vi "Unpack Control Mouse Enter.vi"(11 "ControlMouseEnterMsg":refnum<class "ControlMouseEnterMsg.lvclass">) -> (2 "Time":u32, 3 "Control Label":string, 5 "Ctl Refnum":refnum<vi>)   [LabVIEW 2015, in "ActorEvents.lvlib" / "ControlMouseEnterMsg.lvclass"]
doc: "<License>\nCopyright © 2017 Composed Systems, LLC | All rights reserved\nwww.composed.io\n\nAuthor: Ethan Stern <ethan.stern@composed.io>\n\nThis software is provided \"AS IS\" WITHOUT WARRANTIES, either express or implied, AND IS FOR EDUCATIONAL PURPOSES ONLY.\n</License>"
uses:
  ControlMouseEnterMsg.lvclass
  ControlMouseEnterMsg.lvclass/ControlMouseEnterMsg.ctl
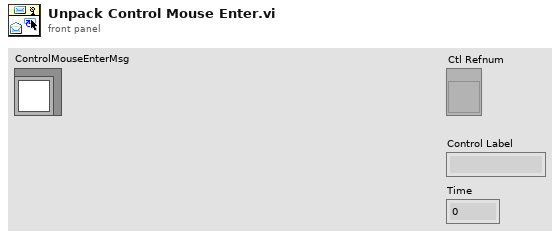
[diagram p1: front panel]
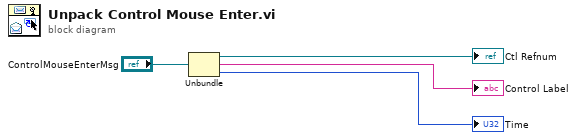
[diagram p0: block diagram]
diagram:
  n1 = Unbundle("ControlMouseEnterMsg") -> (→"Ctl Refnum":refnum<vi>, →"Control Label":string, →"Time":u32)
